vi "SBML_Units_Def.vi"(8 "error in (no error)":errorcluster, 11 "Input SBML File":string) -> (0 "error out":errorcluster, 2 "Units Definition":string[][](table), 3 "Units_Cnt":i32)   [LabVIEW 2014]
doc: "This VI extract the information of species present in SBML file. It takes the complete SBML file as input, and outputs: \nSp_Cnt --> How many species are there\nS_Id_Arr --> Array of species\nSp_Name --> Array containing the name of species\nSp_Init_Amnt --> Array containing the initial amount of species\n\nDesigned by HB\nhaba@dtu.dk"
panel:
  out "Units_Kind":string[](array[string])
  out "Units_Value":string[](array[string])
  out "Units_Name":string[](array[string])
  out "Units_ID":string[](array[string])
  out "List of Units":string
  # "Names"
  # "Initial Amount"
  # "ID"
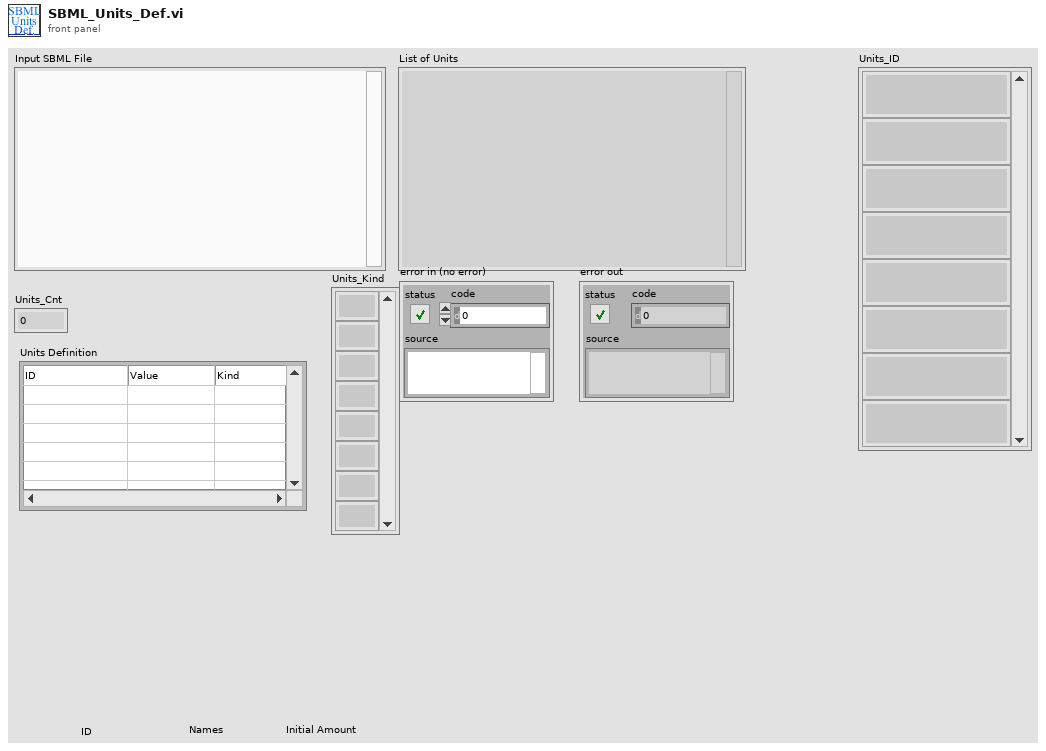
[diagram p1: front panel]
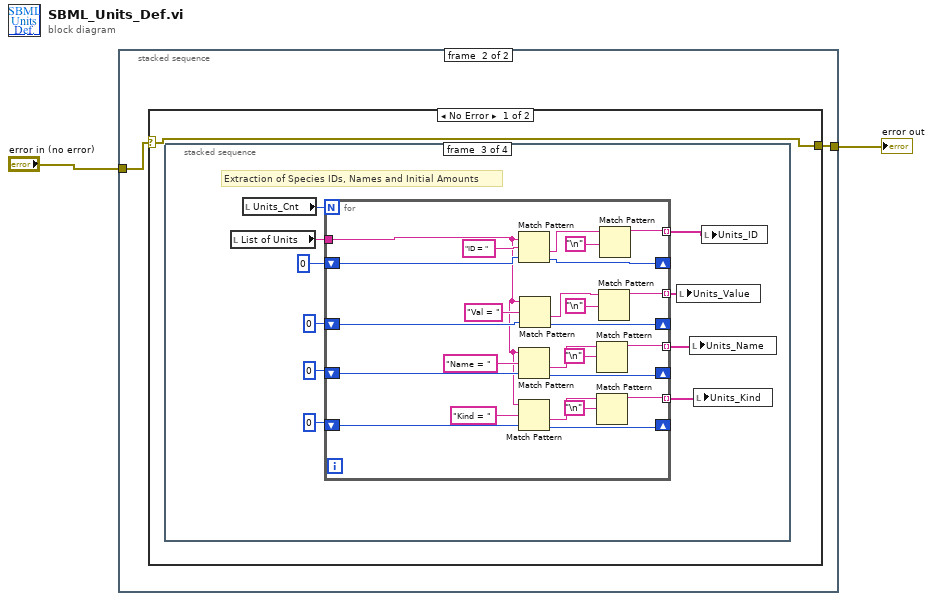
[diagram p0: block diagram]
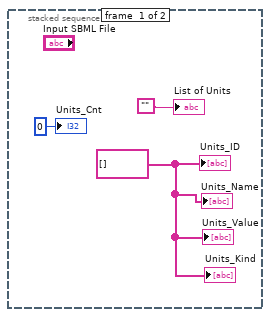
[diagram p2: hidden frame]
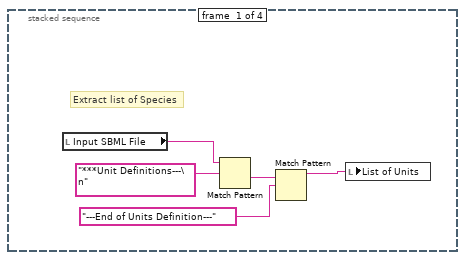
[diagram p3: hidden frame]
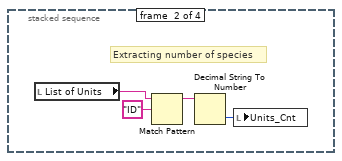
[diagram p4: hidden frame]
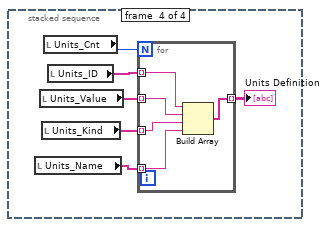
[diagram p5: hidden frame]
diagram:
  n1 = stacked-sequence {
    tunnel: "error in (no error)" -> [_ w6]
    tunnel: [_ w7] -> w1
    frame #0 {
      w3 = string[] [] ("Sp_Id_Arr")
      "List of Units" <- "" ("Full SBML File")
      "Units_Cnt" <- 0 ("Sp_cnt")
      "Units_ID" <- w3
      "Units_Name" <- w3
      "Units_Value" <- w3
      "Units_Kind" <- w3
    }
    frame #1 {
      n2 = case shown="No Error" w6 {
        selector: w6 -> [w8 w64]
        tunnel: [w8 w64] -> w7
        frame No Error {
          n3 = stacked-sequence {
            frame #0 {
              # "Extract list of Species"
              n4 = local read "Input SBML File"() -> (w10:string)
              n5 = Match Pattern(string=w10, regular expression="***Unit Definitions---\n") -> (after substring=w12:string)  [unwired: 1 in, 3 out]
              n6 = Match Pattern(string=w12, regular expression="---End of Units Definition---") -> (before substring=w9:string)  [unwired: 1 in, 3 out]
              n7 = local write "List of Units"(w9) -> ()
            }
            frame #1 {
              # "Extracting number of species"
              n8 = local read "List of Units"() -> (w14:string)
              n9 = Match Pattern(string=w14, regular expression="ID") -> (before substring=w16:string)  [unwired: 1 in, 3 out]
              n10 = Decimal String To Number(string=w16) -> (number=w15:i32)  [unwired: 2 in, 1 out]
              n11 = local write "Units_Cnt"(w15) -> ()
            }
            frame #2 {
              # "Extraction of Species IDs, Names and Initial Amounts"
              n12 = local read "List of Units"() -> (w25:string)
              n13 = local read "Units_Cnt"() -> (w24:i32)
              n14 = for {
                N: w24 -> [_]
                tunnel: w25 -> [w28]
                shift-right: [w49] -> _
                shift-left: 0 ("offset past match") -> [w48]
                shift-right: [w44] -> _
                shift-left: 0 ("offset past match") -> [w43]
                tunnel: [w42] -> w23 mode=indexing
                tunnel: [w41] -> w22 mode=indexing
                shift-right: [w39] -> _
                shift-left: 0 ("offset of match") -> [w40]
                tunnel: [w38] -> w20 mode=indexing
                shift-right: [w30] -> _
                shift-left: 0 ("offset of match") -> [w29]
                tunnel: [w31] -> w19 mode=indexing
                n15 = Match Pattern(string=w28, regular expression="ID = ", offset (0)=w43) -> (after substring=w45:string, offset past match=w44:i32)  [unwired: 2 out]
                n16 = Match Pattern(string=w28, regular expression="Name = ", offset (0)=w40) -> (after substring=w37:string, offset past match=w39:i32)  [unwired: 2 out]
                n17 = Match Pattern(string=w28, regular expression="Kind = ", offset (0)=w29) -> (after substring=w32:string, offset past match=w30:i32)  [unwired: 2 out]
                n18 = Match Pattern(string=w28, regular expression="Val = ", offset (0)=w48) -> (after substring=w52:string, offset past match=w49:i32)  [unwired: 2 out]
                n19 = Match Pattern(string=w37, regular expression="\n") -> (before substring=w38:string)  [unwired: 1 in, 3 out]
                n20 = Match Pattern(string=w32, regular expression="\n") -> (before substring=w31:string)  [unwired: 1 in, 3 out]
                n21 = Match Pattern(string=w52, regular expression="\n") -> (before substring=w42:string)  [unwired: 1 in, 3 out]
                n22 = Match Pattern(string=w45, regular expression="\n") -> (before substring=w41:string)  [unwired: 1 in, 3 out]
              }
              n23 = local write "Units_Value"(w23) -> ()
              n24 = local write "Units_Name"(w20) -> ()
              n25 = local write "Units_Kind"(w19) -> ()
              n26 = local write "Units_ID"(w22) -> ()
            }
            frame #3 {
              n27 = local read "Units_Name"() -> (w55:string[])
              n28 = local read "Units_Value"() -> (w57:string[])
              n29 = local read "Units_Kind"() -> (w53:string[])
              n30 = local read "Units_Cnt"() -> (w56:i32)
              n31 = local read "Units_ID"() -> (w58:string[])
              n32 = for {
                N: w56 -> [_]
                tunnel: w58 -> [w63] mode=indexing
                tunnel: w57 -> [w62] mode=indexing
                tunnel: [w61] -> w54 mode=indexing
                tunnel: w55 -> [w60] mode=indexing
                tunnel: w53 -> [w59] mode=indexing
                n33 = Build Array(w63, w62, w59, w60) -> (w61:string[])
              }
              "Units Definition" <- w54
            }
          }
        }
        frame Error {
        }
      }
    }
  }
  "error out" <- w1
